vi "Lvi Subsystem Stop.vi"(8 "error in (no error)":errorcluster, 10 "FinishBuffer":bool, 11 "TaskRef":i32) -> (0 "error out":errorcluster, 2 "function return":u32(ring), 3 "TaskRef out":i32)   [LabVIEW 2022 SP3, in "DtLvLink.lvlib"]
doc: "Calls directly into the entry points of the DLL of the Data Acq SDK to explicitly stop the task. This VI is used by the higher-level VI, DtOLStop."
uses:
  DtLvLink.lvlib
  <userlib>/LV-Link3/DtLvLink_64.dll
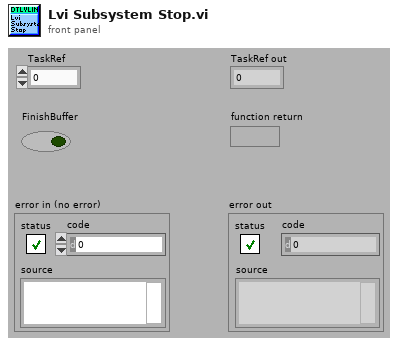
[diagram p1: front panel]
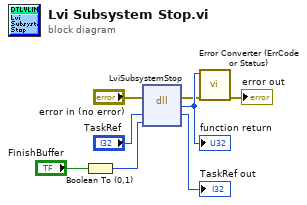
[diagram p0: block diagram]
diagram:
  n1 = Boolean To (0,1)(Boolean="FinishBuffer") -> (0, 1=w4:i16)
  n2 = dll-call lib="C:/Program Files/National Instruments/LabVIEW 2022/user.lib/LV-Link3/DtLvLink_64.*" fn="LviSubsystemStop"(error in="error in (no error)", "TaskRef"="TaskRef", "FinishBuffer"=w4) -> (error out=w2:errorcluster, w8:u32, "TaskRef"=→"TaskRef out":i32)  [unwired: 3 in, 1 out]
  "function return" <- w8
  n3 = call "Error Converter (ErrCode or Status).vi"("error in (no error)"=w2, "error code"=w8) -> ("error out"=→"error out":errorcluster)  [unwired: 9 in]
